vi "Delete UI Reference Mal.vi"(8 "error in (no error)":errorcluster, 10 "Panel":string, 11 "UI Reference Wrapper in":refnum<class "UI Reference Wrapper.lvclass">) -> (0 "error out":errorcluster, 1 "VI Refnum":refnum<vi>, 2 "key not found?":bool, 3 "UI Reference Wrapper out":refnum<class "UI Reference Wrapper.lvclass">)   [LabVIEW 2020, in "UI Reference Wrapper.lvclass"]
uses:
  UI Reference Wrapper.lvclass
  UI Reference Wrapper.lvclass/UI Reference Wrapper.ctl
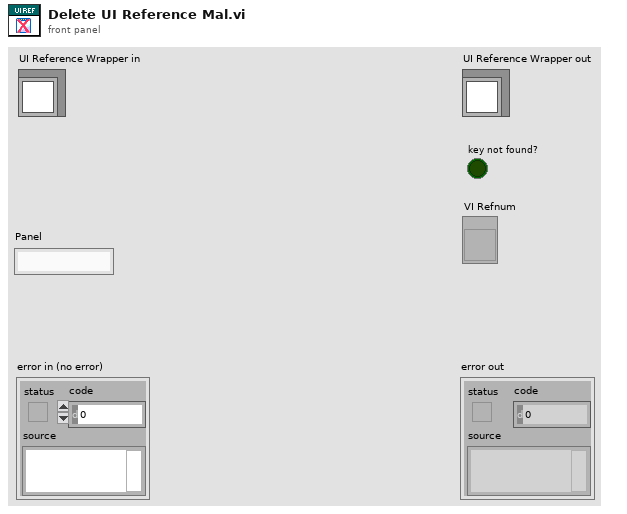
[diagram p1: front panel]
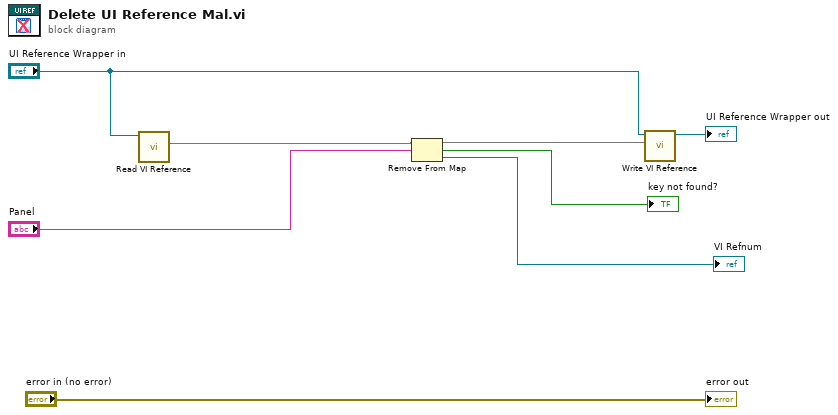
[diagram p0: block diagram]
diagram:
  n1 = call "Read VI Reference.vi"("UI Reference Wrapper in"="UI Reference Wrapper in") -> ("VI Reference Wrappers"=w5:map{string, refnum<vi>})  [unwired: 8 in, 2 out]
  n2 = Remove From Map(10:"Panel", 11:w5) -> (1:→"VI Refnum":refnum<vi>, 2:→"key not found?":bool, 3:w3:map{string, refnum<vi>})
  n3 = call "Write VI Reference.vi"("VI Reference Wrappers"=w3, "UI Reference Wrapper in"="UI Reference Wrapper in") -> ("UI Reference Wrapper out"=→"UI Reference Wrapper out":refnum<class "UI Reference Wrapper.lvclass">)  [unwired: 8 in, 1 out]
  "error out" <- "error in (no error)"
